vi "Scan demo.vi"() -> ()   [LabVIEW 2015]
uses:
  <vilib>/Platform/TimedLoop/XDataNode/timing_clust.ctl
  <vilib>/Platform/TimedLoop/XDataNode/nitl_modes.ctl
  <vilib>/Platform/TimedLoop/XDataNode/wakeup.ctl
  <vilib>/rvi/Emulation/niFpgaSctlEmulationGetInTimedLoop.vi
  Globals.vi
  <vilib>/rvi/Emulation/niFpgaProcessEmulError.vi
  <vilib>/rvi/Emulation/niFpgaEmulationReportErrorSimple.vi
  <vilib>/rvi/Emulation/niFpgaGetClockAttributes.vi
  <vilib>/rvi/Emulation/niFpgaCriticalErrorInLSC.vi
  <vilib>/Platform/TimedLoop/XDataNode/XDataNode.xnode
  <vilib>/Platform/TimedLoop/XDataNode/XDNodeRunTimeDep.lvlib
panel:
  out "WD done":bool=TRUE
  out "大小":i32
  out "数组":u16[](array[numeric])
  out "time":u32
  out "Points read":i16
  out "Output size":i16
  out "Ticks passed":u32
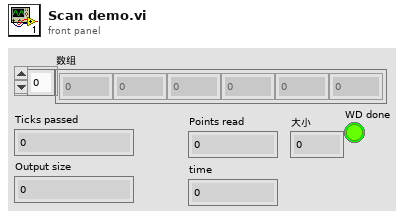
[diagram p1: front panel]
types:
  T1 = typedef "XDNodeRunTimeDep.lvlib/timing_clust.ctl" = cluster{"Expected End [f-1]":u64, "Actual End [f-1]":u64, "Finished Late? [f-1]":bool, "Expected End [i-1]":u64, "Actual End [i-1]":u64, "Finished Late? [i-1]":bool, "Expected Start [i]":u64, "Actual Start [i]":u64, "Expected Start [f]":u64, "Actual Start [f]":u64, "Source Name":string, "Structure Name":string, "Period":i64, "Deadline":i64, "Offset":i64, "Start":i64, "Priority":i32, "Timeout":i32, "Mode":T2, "Wakeup Reason":T3, "Error":errorcluster, "Source Type":string, "Secondary Source Type":string, "Global End Time":u64, "Global Start Time":u64, "Frame Duration":u64, "Iteration Duration":u64, "Assigned CPU":i32, "I/O Scan Engine Mode":u32}
  T2 = typedef "XDNodeRunTimeDep.lvlib/nitl_modes.ctl" = enum32{"No Change", "Process missed periods, maintain original phase", "Discard missed periods, maintain original phase", "Process missed periods, ignore original phase", "Discard missed periods, ignore original phase"}
  T3 = typedef "XDNodeRunTimeDep.lvlib/wakeup.ctl" = enum32{"Normal", "Aborted", "Asynchronous wakeup", "Timing source error", "Timed loop error", "Timeout"}
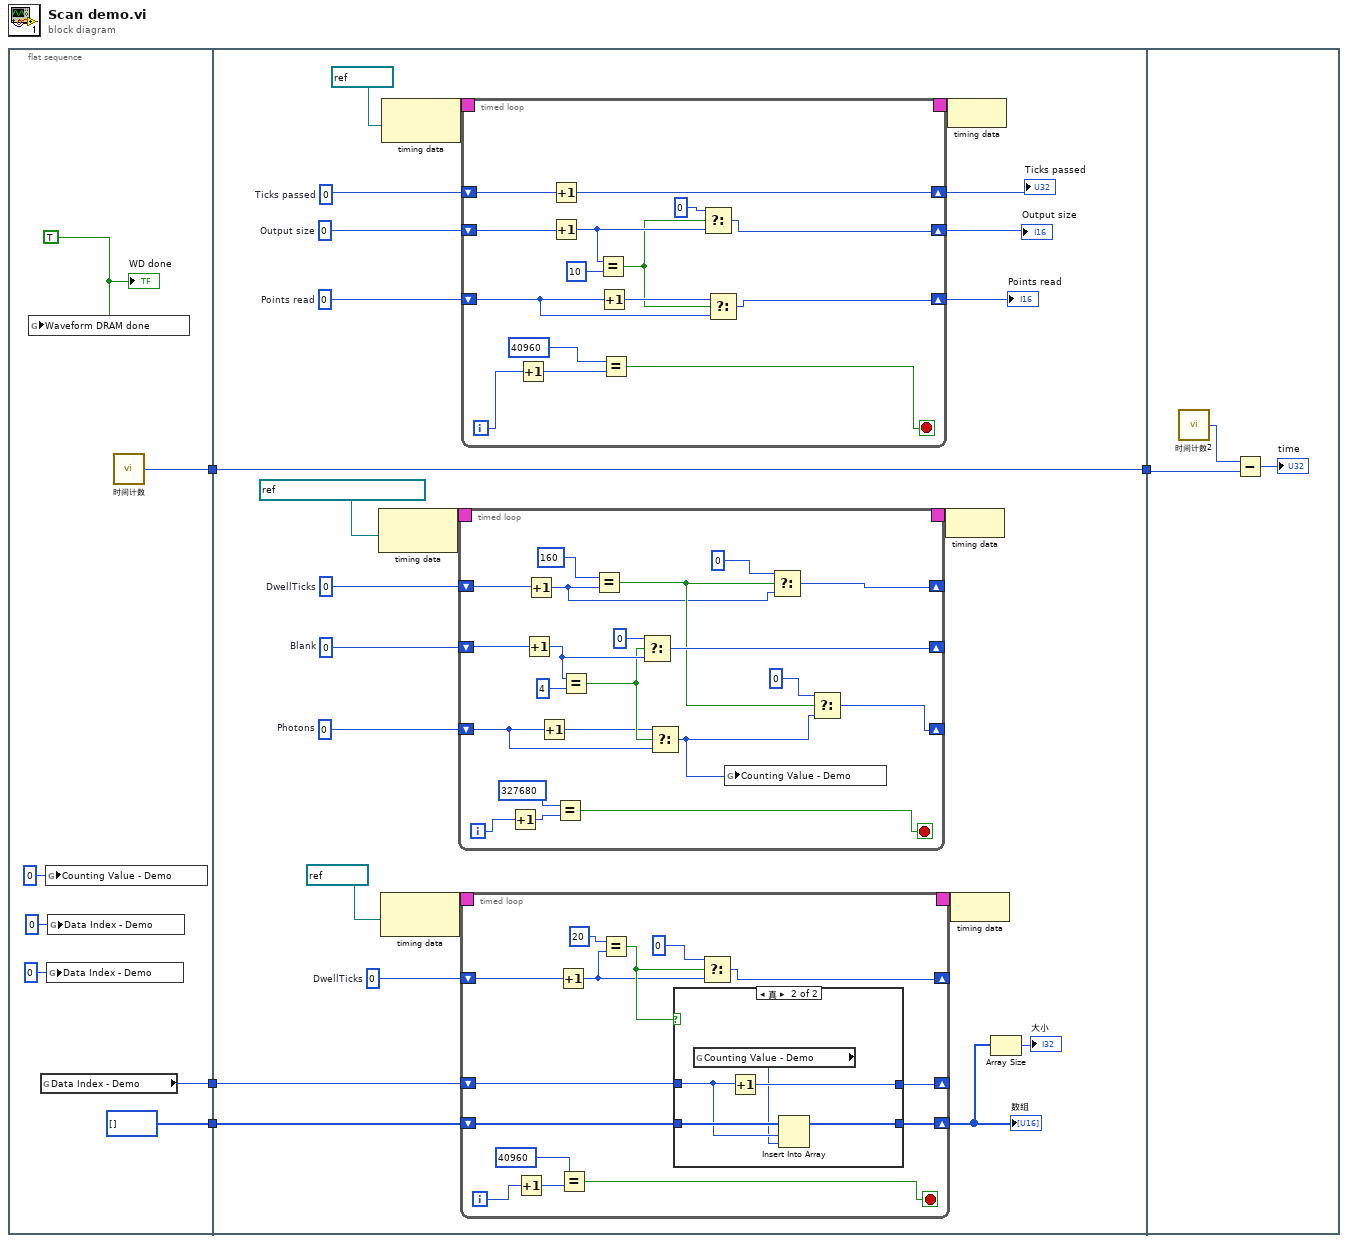
[diagram p0: block diagram]
diagram:
  n1 = flat-sequence {
    tunnel: [w11] -> w4
    tunnel: [u16[] []] -> w2
    tunnel: [w9] -> w1
    tunnel: w4 -> [w26]
    tunnel: [w26] -> w3
    tunnel: w2 -> [w16]
    tunnel: w1 -> [w15]
    tunnel: w3 -> [w112]
    frame #0 {
      w5 = TRUE
      n2 = global write "Globals.vi" "Waveform DRAM done"(w5) -> ()
      n3 = global read "Globals.vi" "Data Index - Demo"() -> (w9:i32)
      n4 = global write "Globals.vi" "Counting Value - Demo"(u16 0 ("Counting Value - Demo")) -> ()
      n5 = global write "Globals.vi" "Data Index - Demo"(0 ("Data Index - Demo")) -> ()
      n6 = global write "Globals.vi" "Data Index - Demo"(0 ("Data Index - Demo")) -> ()
      n7 = call "时间计数"() -> ("Tick Count(uSec)"=w11:u32)
      "WD done" <- w5
    }
    frame #1 {
      w14 = u32 0  # DwellTicks
      w18 = u32 0  # DwellTicks
      w21 = u16 0  # Photons
      w22 = i16 0  # Blank
      w30 = i16 0  # Points read
      w31 = i16 0  # Output size
      w32 = u32 0  # Ticks passed
      n8 = node-c288(refnum<k21> "40 MHz Onboard Clock" ("源名称")) -> (w25:T1)
      n9 = node-c288(refnum<k21> "5MHz" ("源名称")) -> (w20:T1)
      n10 = node-c288(refnum<k21> "5MHz" ("源名称")) -> (w35:T1)
      n11 = timed-loop {
        timing: w25 -> [_]
        timing-out: [_] -> w24
        shift-right: [w80] -> _
        shift-left: w22 -> [w83]
        shift-right: [w75] -> _
        shift-left: w21 -> [w76]
        shift-right: [w67] -> _
        shift-left: w14 -> [w72]
        i -> [w65]
        stop <- w63 stop-if-true
        n12 = Increment(x=w65) -> (x+1=w66:i32)
        n13 = Increment(x=w83) -> (x+1=w81:i16)
        n14 = Increment(x=w72) -> (x+1=w69:u32)
        n15 = Increment(x=w76) -> (x+1=w77:u16)
        n16 = Equal?(x=327680, y=w66) -> (x = y?=w63:bool)
        n17 = Equal?(x=w81, y=i16 4) -> (x = y?=w78:bool)
        n18 = Equal?(x=u32 160, y=w69) -> (x = y?=w70:bool)
        n19 = Select(t=i16 0, s=w78, f=w81) -> (s? t:f=w80:i16)
        n20 = Select(t=w77, s=w78, f=w76) -> (s? t:f=w73:u16)
        n21 = global write "Globals.vi" "Counting Value - Demo"(w73) -> ()
        n22 = Select(t=u32 0, s=w70, f=w69) -> (s? t:f=w67:u32)
        n23 = Select(t=u16 0, s=w70, f=w73) -> (s? t:f=w75:u16)
      }
      n24 = timed-loop {
        timing: w20 -> [_]
        timing-out: [_] -> w19
        shift-right: [w47] -> _
        shift-left: w18 -> [w45]
        shift-right: [w41] -> _
        shift-left: w15 -> [w42]
        shift-right: [w40] -> w13
        shift-left: w16 -> [w43]
        i -> [w39]
        stop <- w36 stop-if-true
        n25 = Increment(x=w39) -> (x+1=w38:i32)
        n26 = Increment(x=w45) -> (x+1=w44:u32)
        n27 = Equal?(x=40960, y=w38) -> (x = y?=w36:bool)
        n28 = Equal?(x=u32 20, y=w44) -> (x = y?=w46:bool)
        n29 = case shown="真" w46 {
          tunnel: w43 -> [w50 w56]
          tunnel: w42 -> [w51 w54]
          tunnel: [w51 w55] -> w41
          tunnel: [w50 w53] -> w40
          frame False {
          }
          frame True {
            n30 = global read "Globals.vi" "Counting Value - Demo"() -> (w52:u16)
            n31 = Increment(x=w54) -> (x+1=w55:i32)
            n32 = Insert Into Array(array=w56, index=w54, new element=w52) -> (w53:u16[])
          }
        }
        n33 = Select(t=u32 0, s=w46, f=w44) -> (s? t:f=w47:u32)
      }
      "数组" <- w13
      n34 = timed-loop {
        timing: w35 -> [_]
        timing-out: [_] -> w34
        shift-right: [w103] -> w29
        shift-left: w32 -> [w104]
        shift-right: [w99] -> w28
        shift-left: w31 -> [w102]
        shift-right: [w96] -> w27
        shift-left: w30 -> [w95]
        i -> [w94]
        stop <- w90 stop-if-true
        n35 = Increment(x=w94) -> (x+1=w92:i32)
        n36 = Increment(x=w104) -> (x+1=w103:u32)
        n37 = Increment(x=w102) -> (x+1=w100:i16)
        n38 = Equal?(x=w100, y=i16 10) -> (x = y?=w91:bool)
        n39 = Increment(x=w95) -> (x+1=w97:i16)
        n40 = Equal?(x=40960, y=w92) -> (x = y?=w90:bool)
        n41 = Select(t=i16 0, s=w91, f=w100) -> (s? t:f=w99:i16)
        n42 = Select(t=w97, s=w91, f=w95) -> (s? t:f=w96:i16)
      }
      "Ticks passed" <- w29
      "Output size" <- w28
      "Points read" <- w27
      n43 = node-c288(w24) -> ()
      n44 = node-c288(w34) -> ()
      n45 = node-c288(w19) -> ()
      n46 = Array Size(array=w13) -> (size(s)=→"大小":i32)
    }
    frame #2 {
      n47 = call "时间计数2"() -> ("Tick Count(uSec)"=w113:u32)
      n48 = Subtract(x=w113, y=w112) -> (x-y=→"time":u32)
    }
  }
